vi "Pre Launch Init.vi"(11 "Digital Reader in":refnum<class "Digital Reader.lvclass">) -> (0 "error out":errorcluster, 3 "Digital Reader out":refnum<class "Digital Reader.lvclass">)   [LabVIEW 2024, in "DAQmx Actor.lvlib" / "Digital Reader.lvclass"]
doc: "<p>(<strong>Filename</strong>: <span class=\"dnl\">Actor Framework.lvlib:Actor.lvclass:Pre Launch Init.vi</span>)</p>\n<p>Defines behavior that occurs after the <a href=\"nihelplauncher://docs/csh?context=lvcore_lvcomm_af_launch_nested_actor\">Launch Nested Actor</a> method is invoked but before the actor's Actor Core method begins running.</p>\n<p>By default, this method does nothing. A descendant class may override it to define behavior.</p>"
uses:
  Digital Reader.lvclass
  Digital Reader.lvclass/Digital Reader.ctl
  DAQmx Actor/DAQmx Actor.lvclass
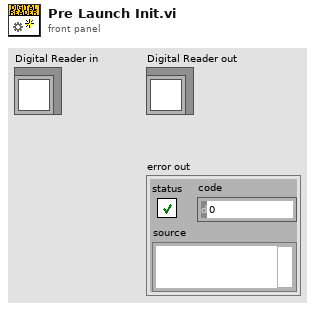
[diagram p1: front panel]
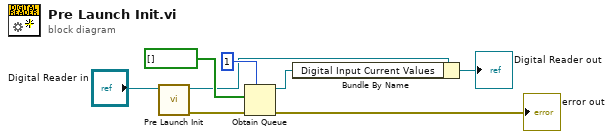
[diagram p0: block diagram]
diagram:
  n1 = call-parent "Pre Launch Init.vi"("DAQmx Actor in"="Digital Reader in") -> ("error out"=w5:errorcluster, "DAQmx Actor out"=w2:refnum<class "Digital Reader.lvclass">)  [unwired: 9 in]
  n2 = Obtain Queue(max queue size (-1, unlimited)=1, element data type=bool[] [], error in (no error)=w5) -> (queue out=w3:refnum<queue>, error out=→"error out":errorcluster)  [unwired: 2 in, 1 out]
  n3 = Bundle By Name(cluster=w2, "Digital Input Current Values"=w3) -> (→"Digital Reader out":refnum<class "Digital Reader.lvclass">)
